vi "Int32ToNode(viaString).vi"(0 "Tree DVR in":refnum<data-value>, 1 "I32 in":i32, 3 "error in (no error)":errorcluster, 4 "NodePath":string) -> (5 "Tree DVR out":refnum<data-value>, 6 "TreeNode DVR out":refnum<data-value>, 7 "error out":errorcluster)   [LabVIEW 2014]
uses:
  <vilib>/MDSplus/Classes/Tree_Class/Tree.lvclass
  <vilib>/MDSplus/Classes/Data_Class/TreeNode_Class/TreeNode.lvclass
  <vilib>/MDSplus/Library/MDSplus.lvlib
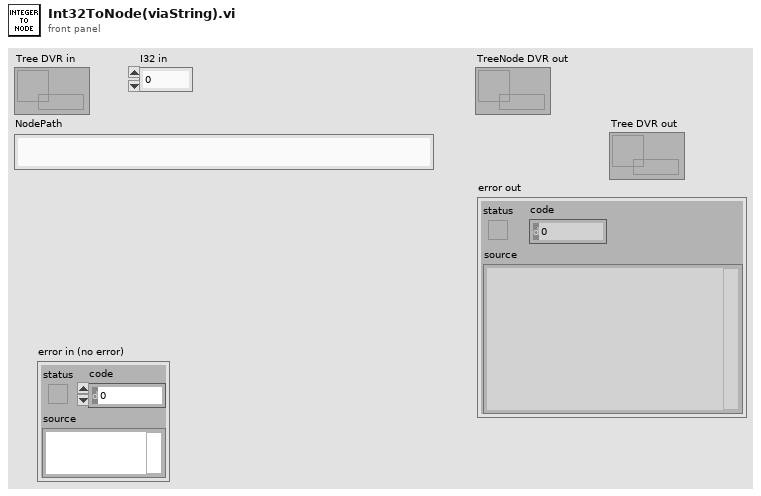
[diagram p1: front panel]
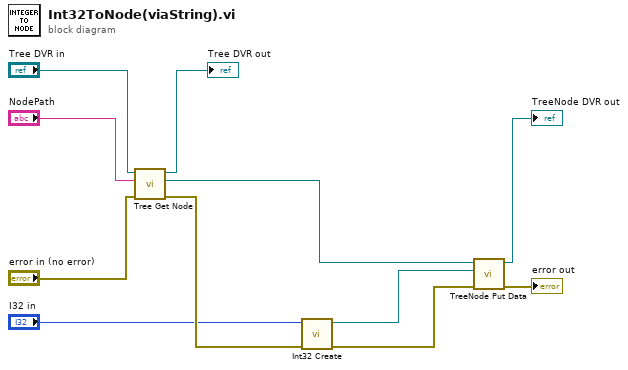
[diagram p0: block diagram]
diagram:
  n1 = call <vilib>:"Tree Get Node.vi"("error in (no error)"="error in (no error)", "Path"="NodePath", "Tree DVR in"="Tree DVR in") -> ("error out"=w8:errorcluster, "Node out"=w11:refnum<data-value>, "Tree DVR out"=→"Tree DVR out":refnum<data-value>)  [unwired: 6 in]
  n2 = call <vilib>:"Int32 Create.vi"("error in (no error)"=w8, "I32 in"="I32 in") -> ("error out"=w9:errorcluster, "Int32 DVR out"=w10:refnum<data-value>)  [unwired: 8 in]
  n3 = call <vilib>:"TreeNode Put Data.vi"("error in (no error)"=w9, "Data"=w10, "TreeNode DVR in"=w11) -> ("error out"=→"error out":errorcluster, "TreeNode DVR out"=→"TreeNode DVR out":refnum<data-value>)  [unwired: 7 in]
